vi "Read Time Params.vi"(8 "error in (no error)":errorcluster, 11 "TX Speed in":refnum<class "TX Speed.lvclass">) -> (0 "error out":errorcluster, 2 "Time Params":T1={"f_SCL(KHz)"=100, "t_HIGH (ns)"=5000, "t_LOW (ns)"=5000, "t_SU;STA (ns)"=4700, "t_HD;STA (ns)"=4000, "t_SU;DAT (ns)"=2500, "t_HD;DAT (ns)"=2500, "t_SU;STO (ns)"=4000, "t_BUF (ns)"=4700} {"t_HIGH (ns)" max=50000 step=1 format="%#.0f"; "t_LOW (ns)" max=50000 step=1 format="%#.0f"; "f_SCL(KHz)" min=10 max=1000 step=1}, 3 "TX Speed out":refnum<class "TX Speed.lvclass">)   [LabVIEW 2020, in "TX Speed.lvclass"]
uses:
  TX Speed.lvclass
  TypeDef/Timing Parameters Cluster.ctl
  TX Speed.lvclass/TX Speed.ctl
  I2C Controller Lib.lvlib
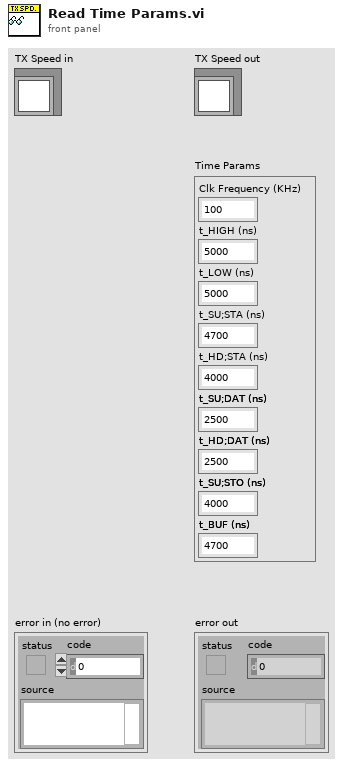
[diagram p1: front panel]
types:
  T1 = typedef "I2C Controller Lib.lvlib/Timing Parameters Cluster.ctl" = cluster{"f_SCL(KHz)":u32, "t_HIGH (ns)":u32, "t_LOW (ns)":u32, "t_SU;STA (ns)":u32, "t_HD;STA (ns)":u32, "t_SU;DAT (ns)":u32, "t_HD;DAT (ns)":u32, "t_SU;STO (ns)":u32, "t_BUF (ns)":u32}
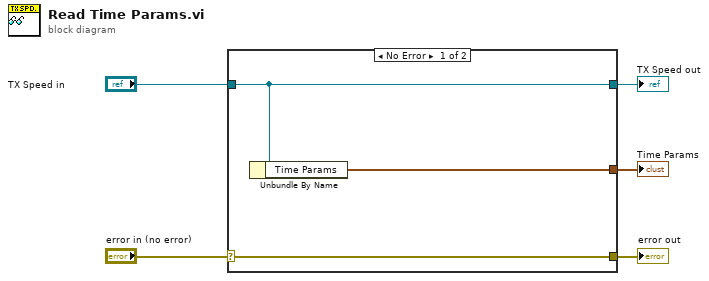
[diagram p0: block diagram]
diagram:
  n1 = case shown="No Error" "error in (no error)" {
    selector: "error in (no error)" -> [w8 w9]
    tunnel: [w8 w9] -> w4
    tunnel: [w7 w10] -> w2
    tunnel: "TX Speed in" -> [w7 w10]
    tunnel: [w6 _] -> w1
    frame No Error {
      n2 = Unbundle By Name(w7) -> ("Time Params"=w6:T1)
    }
    frame Error {
    }
  }
  "error out" <- w4
  "TX Speed out" <- w2
  "Time Params" <- w1
